vi "UpdateConfiguration.vi"(0 "reference in":refnum<class "Control.lvclass">, 2 "FP Configuration":T1, 5 "error in (no error)":errorcluster) -> (14 "reference out":refnum<class "Control.lvclass">, 19 "error out":errorcluster)   [LabVIEW 2014, in "FrontPanelPublisher.lvlib" / "Control.lvclass"]
uses:
  Control.lvclass
  WebFrontPanel_class/Controls/FPObjectConfiguration.ctl
  Object_class/Object.lvclass
  FrontPanelPublisher.lvlib
  WebFrontPanel_class/WebFrontPanel.lvclass
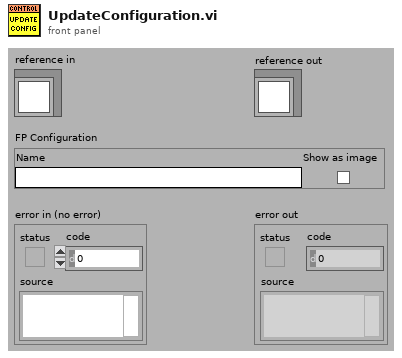
[diagram p1: front panel]
types:
  T1 = typedef "FrontPanelPublisher.lvlib/WebFrontPanel.lvclass/FPObjectConfiguration.ctl" = cluster{"Name":string, "Show as image":bool}
  T2 = typedef "FrontPanelPublisher.lvlib/Control.lvclass/Attributes.ctl" = cluster{"Description":string, "Indicator":bool, "Default Value":variant, "Control Index":i32, "Label":refnum<class "Text.lvclass">, "Caption":refnum<class "Text.lvclass">, "Use Picture":bool, "Image1 b64":string, "Image2 b64":string}
  T3 = typedef "FrontPanelPublisher.lvlib/Object.lvclass/Attributes.ctl" = cluster{"UID":i32, "Type":string, "Coordinates":T4, "Reference":refnum<vi>}
  T4 = typedef "FrontPanelPublisher.lvlib/Object.lvclass/Coordinates.ctl" = cluster{"Left":i32, "Top":i32, "Height":u32, "Width":u32}
  T5 = typedef "LVRectTypeDef.ctl" = cluster{"Left":i16, "Top":i16, "Right":i16, "Bottom":i16}
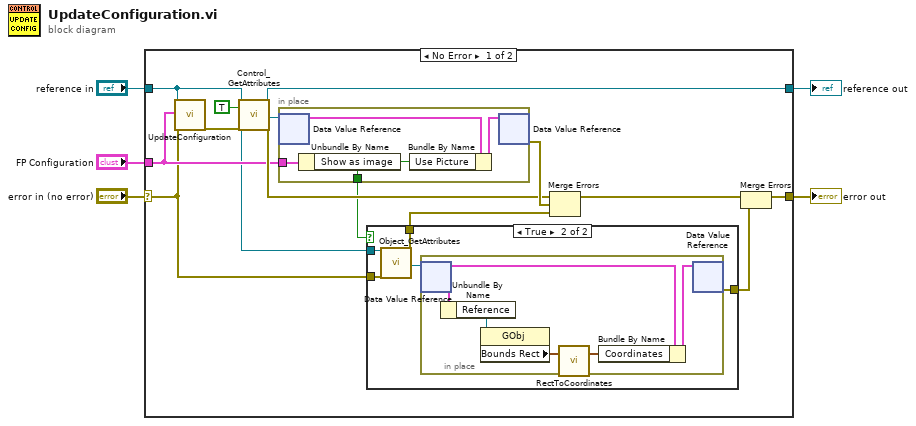
[diagram p0: block diagram]
diagram:
  n1 = case shown="No Error" "error in (no error)" {
    selector: "error in (no error)" -> [w10 w36]
    tunnel: [w6 w36] -> w4
    tunnel: [w18 w35] -> w2
    tunnel: "reference in" -> [w11 w35]
    tunnel: "FP Configuration" -> [w13 _]
    frame No Error {
      n2 = call-parent "UpdateConfiguration.vi"("reference in"=w11, "FP Configuration"=w13, "error in (no error)"=w10) -> ("error out"=w14:errorcluster)  [unwired: 15 in, 1 out]
      n3 = call "Control_GetAttributes.vi"("reference in"=w11, "OnlyGetDvrReference(False)"=TRUE, "error in (no error)"=w14) -> ("reference out"=w18:refnum<class "Control.lvclass">, "DataRef"=w17:refnum<data-value>, "error out"=w15:errorcluster)  [unwired: 13 in, 1 out]
      n4 = in-place {
        in-place-border: w13 -> [w32]
        in-place-border: [w31] -> w12
        n5 = in-place-dvr #1(w17) -> (w33:T2)  [unwired: 1 out]
        n6 = Unbundle By Name(w32) -> ("Show as image"=w31:bool)
        n7 = Bundle By Name(cluster=w33, "Use Picture"=w31) -> (w34:T2)
        n8 = in-place-dvr #1(w34) -> (w19:errorcluster)  [unwired: 1 out]
      }
      n9 = case shown="True" w12 {
        tunnel: w11 -> [_ w24]
        tunnel: w10 -> [w20 w23]
        tunnel: [w20 w22] -> w9
        tunnel: [w20 w21] -> w8
        frame False {
        }
        frame True {
          n10 = call "Object_GetAttributes.vi"("reference in"=w24, "error in (no error)"=w23) -> ("DataRef"=w25:refnum<data-value>, "error out"=w22:errorcluster)  [unwired: 14 in, 2 out]
          n11 = in-place {
            n12 = in-place-dvr #2(w25) -> (w27:T3)  [unwired: 1 out]
            n13 = Unbundle By Name(w27) -> ("Reference"=w28:refnum<vi>)
            n14 = property class="GObj"(reference=w28) -> ("Bounds Rect"=w30:T5)  [unwired: 1 in, 2 out]
            n15 = call "RectToCoordinates.vi"("Rect"=w30) -> ("Coordinates"=w29:T4)  [unwired: 2 in]
            n16 = Bundle By Name(cluster=w27, "Coordinates"=w29) -> (w26:T3)
            n17 = in-place-dvr #2(w26) -> (w21:errorcluster)  [unwired: 1 out]
          }
        }
      }
      n18 = Merge Errors(w15, w19, w9) -> (w7:errorcluster)
      n19 = Merge Errors(w7, w8) -> (w6:errorcluster)
    }
    frame Error {
    }
  }
  "error out" <- w4
  "reference out" <- w2
